vi "GE 5565PIORC.DMA.Is Done.vi"(8 "error in (no error)":errorcluster, 11 "GE 5565PIORC in":refnum<class "GE 5565PIORC.lvclass">) -> (0 "error out":errorcluster, 2 "done?":bool, 3 "GE 5565PIORC out":refnum<class "GE 5565PIORC.lvclass">)   [LabVIEW 2016, in "GE 5565PIORC.lvclass"]
doc: "Checks the DMA Inactive register to see if the DMA transfer is complete."
uses:
  GE 5565PIORC.lvclass
  GE 5565PIORC.lvclass/GE 5565PIORC.ctl
  Properties/Registers/GE 5565PIORC.Registers.Local Configuration.Read.vi
  Properties/Registers/GE 5565PIORC.Registers.Local Configuration.Read (U8).vi
  GE 5565PIORC.Bit Manipulation.Get Bit.vi
  GE 5565PIORC.Bit Manipulation.Get Bit (U8).vi
  GE 5565PIORC.Registers.Read.vi
  GE 5565PIORC.Registers.Read (U8).vi
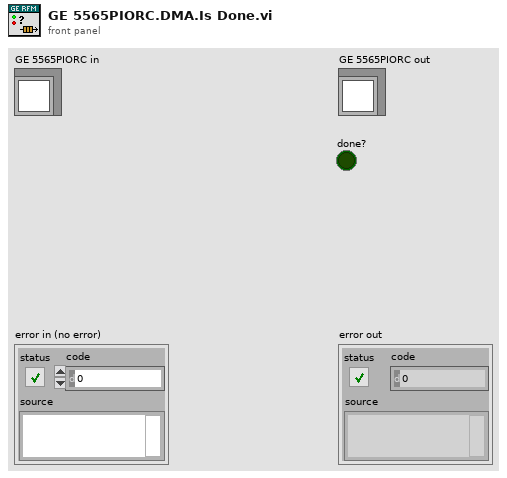
[diagram p1: front panel]
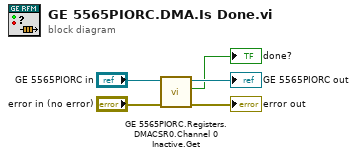
[diagram p0: block diagram]
diagram:
  n1 = call "GE 5565PIORC.Registers.DMACSR0.Channel 0 Inactive.Get.vi"("error in (no error)"="error in (no error)", "GE 5565PIORC in"="GE 5565PIORC in") -> ("error out"=→"error out":errorcluster, "Channel 0 Inactive"=→"done?":bool, "GE 5565PIORC out"=→"GE 5565PIORC out":refnum<class "GE 5565PIORC.lvclass">)  [unwired: 7 in]
